vi "IPS120_setpt_rate_chk.vi"(1 "Set Rate":dbl, 2 "Set Point":dbl) -> (0 "chk set pt and rate":bool)   [LabVIEW 2012]
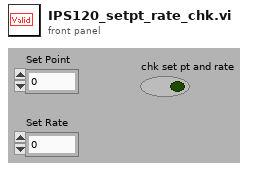
[diagram p1: front panel]
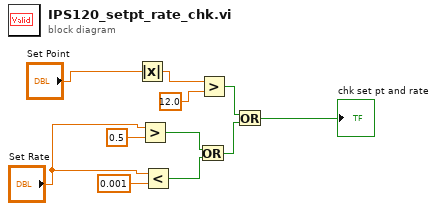
[diagram p0: block diagram]
diagram:
  n1 = Absolute Value(x="Set Point") -> (abs(x)=w2:dbl)
  n2 = Greater?(x="Set Rate", y=0.5) -> (0:w7:bool)
  n3 = Less?(x="Set Rate", y=0.001) -> (x < y?=w8:bool)
  n4 = Or(x=w7, y=w8) -> (x .or. y?=w10:bool)
  n5 = Greater?(x=w2, y=12.0 ("x")) -> (0:w9:bool)
  n6 = Or(x=w9, y=w10) -> (x .or. y?=→"chk set pt and rate":bool)
